vi "Timer - Copie.vi"(0 "index":u32, 1 "Timings in":dbl[][](array[numeric])=[[1578480041.0, 7657.0]], 3 "t1":u32, 4 "t2":u32) -> (2 "Timings out":dbl[][](array[numeric])=[[1578480041.0, 7657.0]])   [LabVIEW 2013]
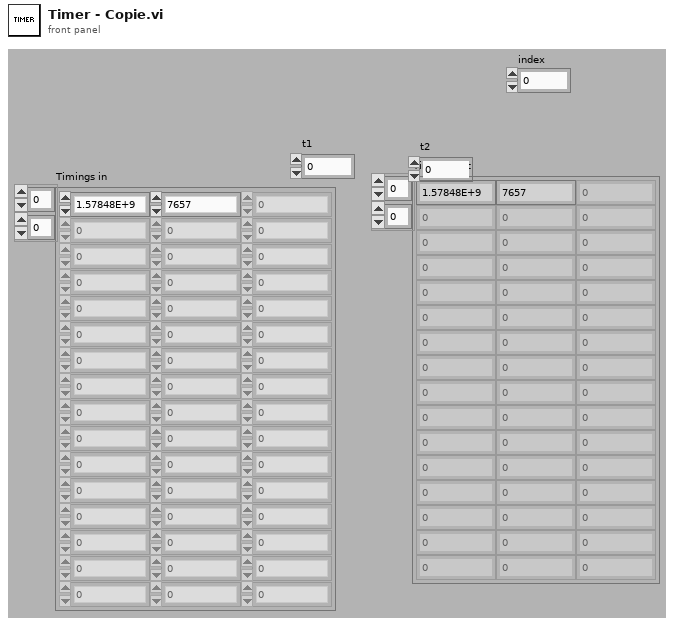
[diagram p1: front panel]
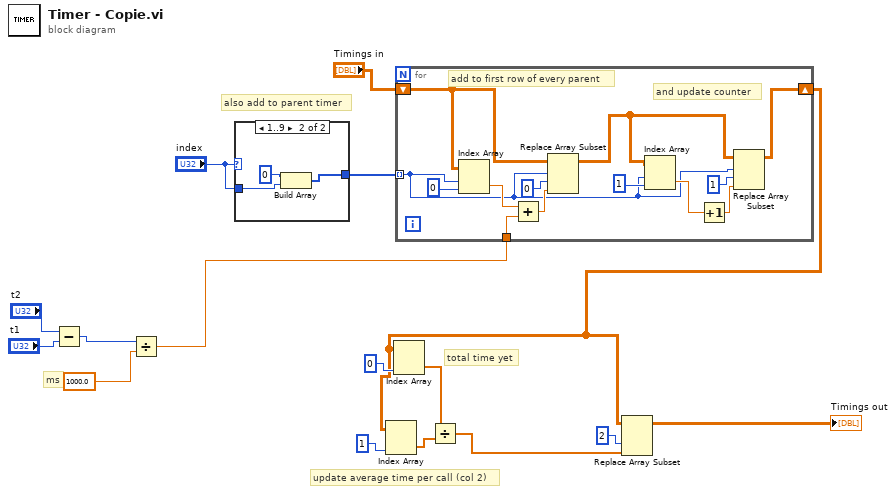
[diagram p0: block diagram]
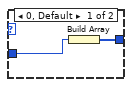
[diagram p2: hidden frame]
diagram:
  # "total time yet"
  # "update average time per call (col 2)"
  # "also add to parent timer"
  # "ms"
  n1 = Subtract(x="t2", y="t1") -> (x-y=w8:u32)
  n2 = Divide(x=w8, y=1000.0) -> (x/y=w13:dbl)
  n3 = case shown="1..9" "index" {
    tunnel: [w18 w19] -> w15
    tunnel: "index" -> [w17 w20]
    frame 0, Default {
      n4 = Build Array(w17) -> (w18:u32[])
    }
    frame 1..9 {
      n5 = Build Array(0, w20) -> (w19:u32[])
    }
  }
  n6 = for {
    tunnel: w15 -> [w22] mode=indexing
    tunnel: w13 -> [w32]
    shift-right: [w29] -> w1
    shift-left: "Timings in" -> [w31]
    # "and update counter"
    # "add to first row of every parent"
    n7 = Index Array(array=w31, index (row)=w22, index (col)=0) -> (element=w33:dbl)
    n8 = Add(x=w33, y=w32) -> (x+y=w34:dbl)
    n9 = Replace Array Subset(array=w31, new element=w34, index (row)=w22, index (col)=0) -> (w28:dbl[][])
    n10 = Index Array(array=w28, index (row)=w22, index (col)=1) -> (element=w30:dbl)
    n11 = Increment(x=w30) -> (x+1=w27:dbl)
    n12 = Replace Array Subset(array=w28, new element=w27, index (row)=w22, index (col)=1) -> (w29:dbl[][])
  }
  n13 = Index Array(array=w1, index (col)=1) -> (element=w2:dbl[])  [unwired: 1 in]
  n14 = Index Array(array=w1, index (col)=0) -> (element=w7:dbl[])  [unwired: 1 in]
  n15 = Divide(x=w7, y=w2) -> (x/y=w6:dbl[])
  n16 = Replace Array Subset(array=w1, new element=w6, index (col)=2) -> (→"Timings out":dbl[][])  [unwired: 1 in]
